vi "ENC-Velocity_Converter.vi"(9 "delta  Encoder Count":i32, 11 "dt (uSec)":u32) -> (0 "Distance (ft)":dbl, 2 "Linear Velocity (ft/s)":dbl, 3 "Rotational Velocity (RPS)":dbl)   [LabVIEW 2015]
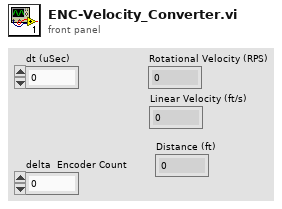
[diagram p1: front panel]
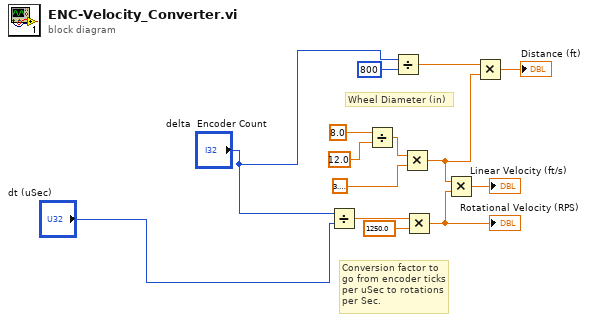
[diagram p0: block diagram]
diagram:
  # "Wheel Diameter (in)"
  # "Conversion factor to \ngo from encoder ticks \nper uSec to rotations\nper Sec."
  n1 = Divide(x="delta  Encoder Count", y="dt (uSec)") -> (x/y=w2:dbl)
  n2 = Divide(x=8.0, y=12.0) -> (x/y=w8:dbl)
  n3 = Divide(x="delta  Encoder Count", y=800) -> (x/y=w12:dbl)
  n4 = Multiply(x=w8, y=3.141592653589793) -> (x*y=w13:dbl)
  n5 = Multiply(x=w2, y=1250.0) -> (x*y=w4:dbl)
  "Rotational Velocity (RPS)" <- w4
  n6 = Multiply(x=w13, y=w4) -> (x*y=→"Linear Velocity (ft/s)":dbl)
  n7 = Multiply(x=w12, y=w13) -> (x*y=→"Distance (ft)":dbl)
